vi "Get Chamber.vi"(8 "error in (no error)":errorcluster, 11 "Instrument.Cryostat in":refnum<class "Instrument.Cryostat.lvclass">) -> (0 "error out":errorcluster, 2 "Status":string, 3 "Instrument.Cryostat out":refnum<class "Instrument.Cryostat.lvclass">)   [LabVIEW 2019, in "Instrument.Cryostat.lvclass"]
uses:
  Instrument.Cryostat.lvclass
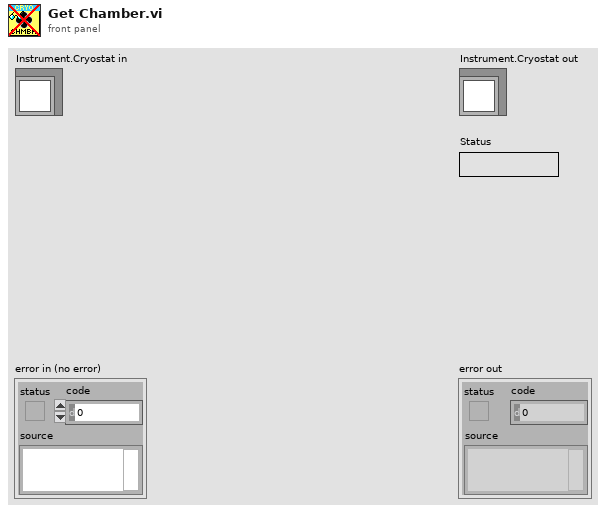
[diagram p1: front panel]
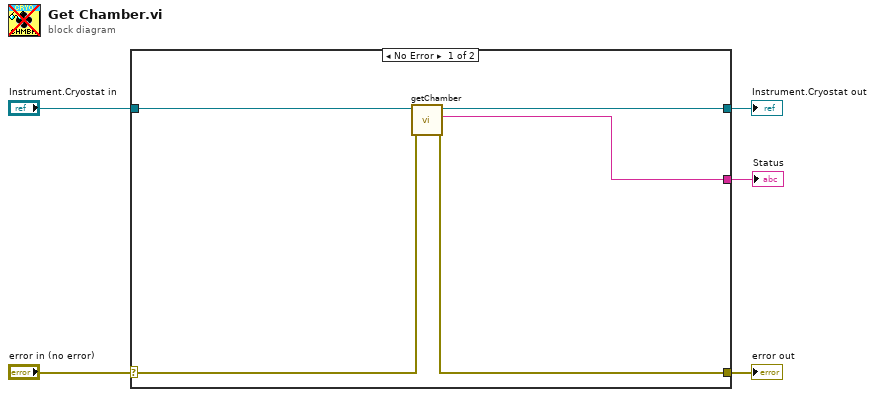
[diagram p0: block diagram]
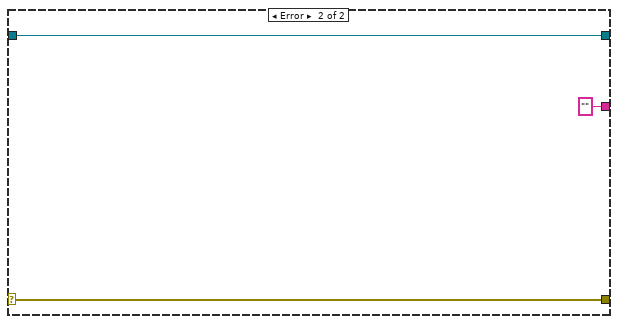
[diagram p2: hidden frame]
diagram:
  n1 = case shown="No Error" "error in (no error)" {
    selector: "error in (no error)" -> [w10 w13]
    tunnel: [w8 w13] -> w4
    tunnel: [w9 w12] -> w2
    tunnel: "Instrument.Cryostat in" -> [w7 w12]
    tunnel: [w6 "" ("Status")] -> w1
    frame No Error {
      n2 = call-dynamic "getChamber.vi"("error in (no error)"=w10, "Instrument.Cryostat in"=w7) -> ("error out"=w8:errorcluster, "Status"=w6:string, "Instrument.Cryostat out"=w9:refnum<class "Instrument.Cryostat.lvclass">)  [unwired: 7 in]
    }
    frame Error {
    }
  }
  "error out" <- w4
  "Instrument.Cryostat out" <- w2
  "Status" <- w1
